vi "Using ParentVIRef If Input Invalid.vi"(7 "VI Ref (calling VI)":refnum<vi>) -> (2 "Using Parent Ref(Need to Destroy)":bool, 3 "VI Ref":refnum<vi>)   [LabVIEW 2017]
doc: "Returns the VI reference wired in, and substitutes the reference of the calling VI when the input reference is invalid. The Using Parent Ref output reports which of the two was used, so the caller knows whether the reference has to be destroyed."
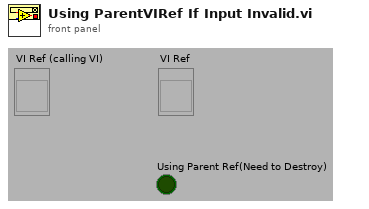
[diagram p1: front panel]
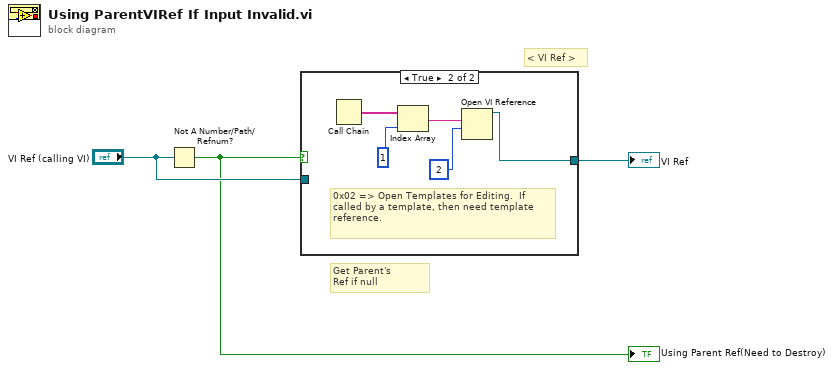
[diagram p0: block diagram]
diagram:
  # "Get Parent's\nRef if null"
  # "< VI Ref >"
  n1 = Not A Number/Path/Refnum?(number/path/refnum="VI Ref (calling VI)") -> (NaN/Path/Refnum?=w1:bool)
  "Using Parent Ref(Need to Destroy)" <- w1
  n2 = case shown="True" w1 {
    tunnel: [w4 w9] -> w2
    tunnel: "VI Ref (calling VI)" -> [w4 _]
    frame False {
    }
    frame True {
      # "0x02 => Open Templates for Editing.  If called by a template, then need template reference."
      n3 = Call Chain() -> (call chain=w5:string[])
      n4 = Index Array(array=w5, index=1 ("Index")) -> (element=w7:string)
      n5 = Open VI Reference(vi path=w7, options=2) -> (vi reference=w9:refnum<vi>)  [unwired: 4 in, 1 out]
    }
  }
  "VI Ref" <- w2
